vi "Remove Quotations.vi"(8 "error in (no error)":errorcluster, 11 "With Quotations":string) -> (0 "error out":errorcluster, 3 "Without Quotations":string)   [LabVIEW 2018, in "ESM303.lvlib" / "ESM303.lvclass"]
uses:
  ESM303.lvclass
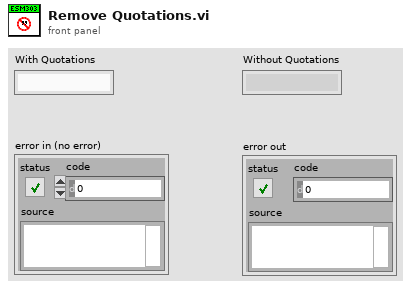
[diagram p1: front panel]
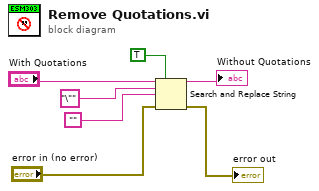
[diagram p0: block diagram]
diagram:
  n1 = Search and Replace String(replace all?=TRUE ("replace all? (F)"), input string="With Quotations", search string="\"", replace string="", error in="error in (no error)") -> (result string=→"Without Quotations":string, error out=→"error out":errorcluster)  [unwired: 3 in, 2 out]
